vi "G# - Polymorphism demo3.vi"() -> ()   [LabVIEW 2020]
doc: "Polymorphism\nThis example shows how objects could be cast to a generic G#Object. It is also possible to treat objects from different class hierarchies the same way. Two G# support methods are also used, \"IsInstanceOf\" that will check if the type is castable and also demo the \"GetClassName\" method. If the reference is castable, the \"MyMethod1\" is executed, else the reference is just closed.\n\nBy using the G# Debugger found in Tools->G# Debugger a text log can be followed showing how the objects were created and destroyed."
uses:
  vi.lib/addons/_AddQ/G#Object/G#Object.lvclass
  DemoClass1_class/DemoClass1.lvclass
  C:/ProjectGSharpDevelopment_2020-3/gsharp/VIPM/Files/vi.lib/addons/_AddQ/G#Object/G#Object.lvclass
  DemoSubClass1_class/DemoSubClass1.lvclass
  DemoSubSubClass1_class/DemoSubSubClass1.lvclass
  AnotherClass_class/AnotherClass.lvclass
panel:
  in  "error in (no error)":errorcluster
  out "IsInstanceOfDemoClass1":bool[](array[boolean])
  out "ClassName":string[](array[string])
  out "error out":errorcluster
  # "Polymorphism\nThis example shows how objects could be cast to a generic G#Object. It is also possible to treat objects from different class hierarchies the same way. Two G# support methods are also used, \"IsInstanceOf\" that will check if the type is castable and also demo the \"GetClassName\" method. If the reference is castable, the \"MyMethod1\" is executed, else the reference is just closed.\n\nBy using the G# Debugger found in Tools->G# Debugger a text log can be followed showing how the objects were created and destroyed."
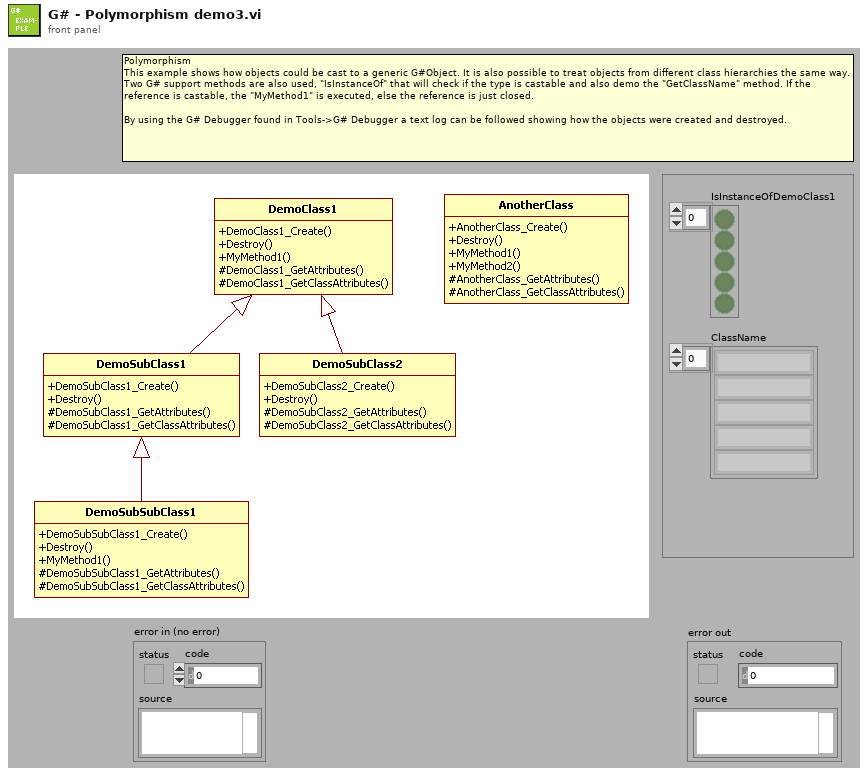
[diagram p1: front panel]
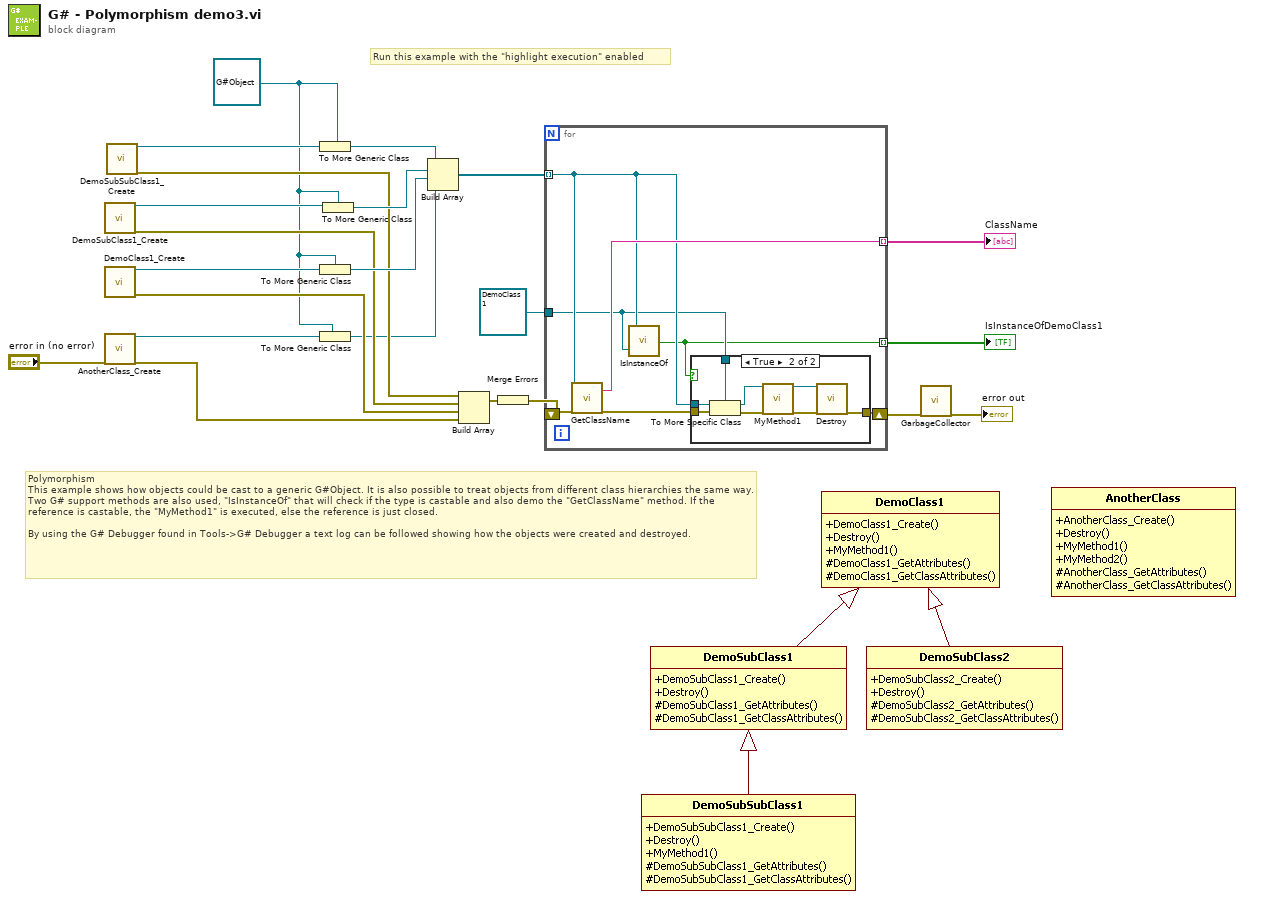
[diagram p0: block diagram]
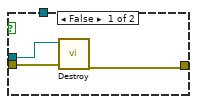
[diagram p2: hidden frame]
diagram:
  w8 = refnum<class "G#Object.lvclass"> refnum ("reference out")
  # "Polymorphism\nThis example shows how objects could be cast to a generic G#Object. It is also possible to treat objects from different class hierarchies the same way. Two G# support methods are also used, \"IsInstanceOf\" that will check if the type is castable and also demo the \"GetClassName\" method. If the reference is castable, the \"MyMethod1\" is executed, else the reference is just closed.\n\nBy using the G# Debugger found in Tools->G# Debugger a text log can be followed showing how the objects were created and destroyed."
  # "Run this example with the \"highlight execution\" enabled"
  n1 = call "DemoSubClass1_Create.vi"() -> ("reference out"=w19:refnum<class "DemoSubClass1.lvclass">, "error out"=w12:errorcluster)  [unwired: 1 in, 17 out]
  n2 = call "DemoClass1_Create.vi"() -> ("reference out"=w18:refnum<class "DemoClass1.lvclass">, "error out"=w11:errorcluster)  [unwired: 1 in, 17 out]
  n3 = call "AnotherClass_Create.vi"("error in (no error)"="error in (no error)") -> ("reference out"=w7:refnum<class "AnotherClass.lvclass">, "error out"=w9:errorcluster)  [unwired: 17 out]
  n4 = call "DemoSubSubClass1_Create.vi"() -> ("reference out"=w20:refnum<class "DemoSubSubClass1.lvclass">, "error out"=w13:errorcluster)  [unwired: 1 in, 17 out]
  n5 = To More Generic Class(target class=w8, reference=w20) -> (generic class reference=w17:refnum<class "G#Object.lvclass">)
  n6 = To More Generic Class(target class=w8, reference=w18) -> (generic class reference=w15:refnum<class "G#Object.lvclass">)
  n7 = To More Generic Class(target class=w8, reference=w7) -> (generic class reference=w6:refnum<class "G#Object.lvclass">)
  n8 = To More Generic Class(target class=w8, reference=w19) -> (generic class reference=w16:refnum<class "G#Object.lvclass">)
  n9 = Build Array(w17, w16, w15, w6) -> (w14:refnum<class "G#Object.lvclass">[])
  n10 = Build Array(w13, w12, w11, w9) -> (w22:errorcluster[])
  n11 = Merge Errors(w22) -> (w21:errorcluster)
  n12 = for {
    tunnel: w14 -> [w26] mode=indexing
    shift-right: [w29] -> w3
    shift-left: w21 -> [w28]
    tunnel: [w27] -> w10 mode=indexing
    tunnel: refnum<class "DemoClass1.lvclass"> refnum ("reference out") -> [w25]
    tunnel: [w23] -> w4 mode=indexing
    n13 = call-dynamic "GetClassName.vi"("reference in"=w26, "error in (no error)"=w28) -> ("class name"=w27:string, "error out"=w24:errorcluster)  [unwired: 13 in, 3 out]
    n14 = call-dynamic "IsInstanceOf.vi"("is object instance of"=w25, "reference in"=w26) -> ("is instance of"=w23:bool)  [unwired: 1 out]
    n15 = case shown="True" w23 {
      tunnel: [w30 w39] -> w29
      tunnel: w26 -> [w31 w35]
      tunnel: w25 -> [_ w34]
      tunnel: w24 -> [w32 w33]
      frame False {
        n16 = call-dynamic "Destroy.vi"("reference in"=w31, "error in (no error)"=w32) -> ("error out"=w30:errorcluster)  [unwired: 16 in, 1 out]
      }
      frame True {
        n17 = To More Specific Class(target class=w34, reference=w35, error in=w33) -> (specific class reference=w36:refnum<class "DemoClass1.lvclass">, error out=w37:errorcluster)
        n18 = call-dynamic "MyMethod1.vi"("reference in"=w36, "error in (no error)"=w37) -> ("reference out"=w38:refnum<class "DemoClass1.lvclass">, "error out"=w40:errorcluster)  [unwired: 16 out]
        n19 = call-dynamic "Destroy.vi"("reference in"=w38, "error in (no error)"=w40) -> ("error out"=w39:errorcluster)  [unwired: 17 out]
      }
    }
  }
  "ClassName" <- w10
  "IsInstanceOfDemoClass1" <- w4
  n20 = call "GarbageCollector.vi"("error in (no error)"=w3) -> ("error out"=→"error out":errorcluster)  [unwired: 16 in, 2 out]
